vi "Initialize Scope and FGEN with Triggering.vi"(10 "FGEN Resources in":refnum<k15>[](array[refnum]), 11 "Scope Resources in":refnum<k15>[](array[refnum])) -> (0 "error out":errorcluster, 2 "FGEN Resources out":refnum<k15>[](array[refnum]), 3 "Scope Resources out":refnum<k15>[](array[refnum]), 5 "scope channels":string[](array[string]))   [LabVIEW 2024]
uses:
  <instrlib>/niFgen/niFgen.llb/niFgen Output Mode.ctl
  <instrlib>/niFgen/niFgen.llb/niFgen Trigger Mode.ctl
  <instrlib>/niScope/Controls/niScope input clock source.ctl
  <instrlib>/niScope/Controls/niScope trigger source digital.ctl
  <instrlib>/niScope/Controls/niScope trigger slope.ctl
  <instrlib>/niScope/Configure/Trigger/niScope Configure Trigger Digital.vi
  <instrlib>/niScope/Controls/niScope trigger source.ctl
  <instrlib>/niScope/Controls/niScope exportable signals.ctl
  <instrlib>/niScope/Controls/niScope export destinations.ctl
  <instrlib>/niScope/Configure/Trigger/niScope Configure Trigger Edge.vi
  <instrlib>/niFgen/niFgen.llb/niFgen_ctl Trigger Source Values (Ring).ctl
  <instrlib>/niFgen/niFgen.llb/niFgen Create Waveform (WDT).vi
  <instrlib>/niFgen/niFgen.llb/niFgen Configure Digital Edge Start Trigger.vi
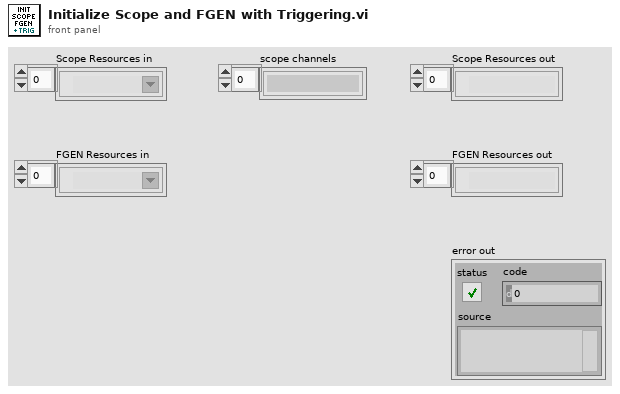
[diagram p1: front panel]
types:
  T1 = typedef "niFgen_ctl Trigger Source Values (Ring).ctl" = string
  T2 = typedef "niScope trigger source digital.ctl" = string
  T3 = typedef "niScope export destinations.ctl" = string
  T4 = typedef "niScope trigger source.ctl" = string
  T5 = typedef "niScope input clock source.ctl" = u16
  T6 = typedef "niScope trigger slope.ctl" = i32
  T7 = typedef "niScope exportable signals.ctl" = u16
  T8 = typedef "niFgen Trigger Mode.ctl" = i32
  T9 = typedef "niFgen Output Mode.ctl" = u32
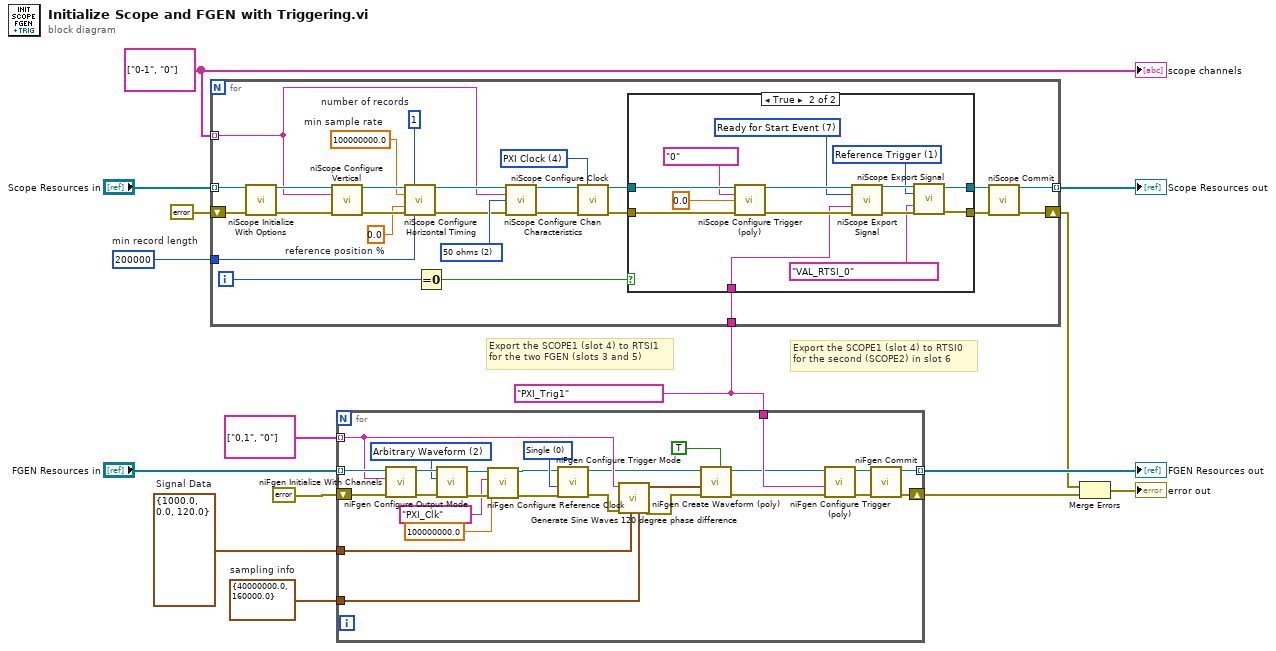
[diagram p0: block diagram]
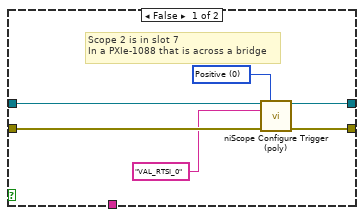
[diagram p2: hidden frame]
diagram:
  w15 = cluster{"f":dbl, "startPhase":dbl, "dPhase":dbl} {"f"=1000.0, "startPhase"=0.0, "dPhase"=120.0}  # Signal Data
  w14 = 200000  # min record length
  w11 = T1 "PXI_Trig1" ("Source")
  w10 = cluster{"Fs":dbl, "#s":dbl} {"Fs"=40000000.0, "#s"=160000.0}  # sampling info
  w6 = string[] ["0-1", "0"] ("channels")
  # "Export the SCOPE1 (slot 4) to RTSI0\nfor the second (SCOPE2) in slot 6"
  # "Export the SCOPE1 (slot 4) to RTSI1\nfor the two FGEN (slots 3 and 5)"
  n1 = for {
    tunnel: "Scope Resources in" -> [w30] mode=indexing
    tunnel: [w36] -> w3 mode=indexing
    tunnel: w6 -> [w17] mode=indexing
    shift-right: [w35] -> w1
    shift-left: errorcluster {"status"=FALSE, "code"=0, "source"=""} ("error out") -> [w34]
    tunnel: w11 -> [w26]
    tunnel: w14 -> [w16]
    i -> [w37]
    w22 = u32 2 items=["1 mega ohm"=0, "50 ohms"=2] ("input impedance")
    w23 = T5 4 items=["None"=0, "RTSI Clock"=1, "PFI 0"=6, "PFI 1"=2, "PFI 2"=3, "PXI Clock"=4, "External"=5, "Clock In"=7] ("input clock source")
    w31 = 0.0  # reference position %
    w32 = 1  # number of records
    w33 = 100000000.0  # min sample rate
    n2 = call <instrlib>:"niScope Initialize With Options.vi"("resource name"=w30, "error in"=w34) -> ("instrument handle"=w41:refnum<k15>, "error out"=w40:errorcluster)  [unwired: 12 in]
    n3 = call <instrlib>:"niScope Configure Vertical.vi"("instrument handle"=w41, "channels"=w17, "error in"=w40) -> ("instrument handle out"=w39:refnum<k15>, "error out"=w38:errorcluster)  [unwired: 11 in]
    n4 = call <instrlib>:"niScope Configure Horizontal Timing.vi"("instrument handle"=w39, "number of records"=w32, "min sample rate"=w33, "reference position"=w31, "error in"=w38, "min record length"=w16) -> ("instrument handle out"=w18:refnum<k15>, "error out"=w19:errorcluster)  [unwired: 8 in]
    n5 = Equal To 0?(x=w37) -> (x = 0?=w29:bool)
    n6 = call <instrlib>:"niScope Configure Chan Characteristics.vi"("instrument handle"=w18, "channels"=w17, "input impedance"=w22, "error in"=w19) -> ("instrument handle out"=w21:refnum<k15>, "error out"=w20:errorcluster)  [unwired: 10 in]
    n7 = call <instrlib>:"niScope Configure Clock.vi"("instrument handle"=w21, "input clock source"=w23, "error in"=w20) -> ("instrument handle out"=w24:refnum<k15>, "error out"=w25:errorcluster)  [unwired: 11 in]
    n8 = case shown="True" w29 {
      tunnel: w25 -> [w47 w60]
      tunnel: [w45 w51] -> w28
      tunnel: [w44 w52] -> w27
      tunnel: w24 -> [w46 w61]
      tunnel: w26 -> [_ w49]
      frame False {
        w42 = T6 0 items=["Positive", "Negative"] ("trigger slope")
        # "Scope 2 is in slot 7\nIn a PXIe-1088 that is across a bridge"
        n9 = call-poly <instrlib>:"niScope Configure Trigger (poly).vi"("instrument handle"=w46, "trigger slope"=w42, "trigger source"=T2 "VAL_RTSI_0", "error in"=w47) -> ("instrument handle out"=w45:refnum<k15>, "error out"=w44:errorcluster)  [unwired: 10 in]
      }
      frame True {
        w50 = T7 1 items=["None"=0, "Start Trigger"=2, "Advance Trigger"=5, "Reference Trigger"=1, "End of Record Event"=4, "End of Acquisition Event"=3, "Ready for Start Event"=7, "Ready for Advance Event"=6, "Ready for Reference Event"=10, "Reference Clock"=100, "Sample Clock"=101, "5 Volt Power"=13] ("signal")
        w55 = T7 7 items=["None"=0, "Start Trigger"=2, "Advance Trigger"=5, "Reference Trigger"=1, "End of Record Event"=4, "End of Acquisition Event"=3, "Ready for Start Event"=7, "Ready for Advance Event"=6, "Ready for Reference Event"=10, "Reference Clock"=100, "Sample Clock"=101, "5 Volt Power"=13] ("signal")
        n10 = call-poly <instrlib>:"niScope Configure Trigger (poly).vi"("instrument handle"=w61, "trigger source"=T4 "0", "trigger level"=0.0, "error in"=w60) -> ("instrument handle out"=w56:refnum<k15>, "error out"=w57:errorcluster)  [unwired: 10 in]
        n11 = call <instrlib>:"niScope Export Signal.vi"("instrument handle"=w56, "signal"=w55, "output terminal"=w49, "error in"=w57) -> ("instrument handle out"=w54:refnum<k15>, "error out"=w53:errorcluster)  [unwired: 10 in]
        n12 = call <instrlib>:"niScope Export Signal.vi"("instrument handle"=w54, "signal"=w50, "output terminal"=T3 "VAL_RTSI_0", "error in"=w53) -> ("instrument handle out"=w51:refnum<k15>, "error out"=w52:errorcluster)  [unwired: 10 in]
      }
    }
    n13 = call <instrlib>:"niScope Commit.vi"("instrument handle"=w28, "error in"=w27) -> ("instrument handle out"=w36:refnum<k15>, "error out"=w35:errorcluster)  [unwired: 12 in]
  }
  "Scope Resources out" <- w3
  n14 = for {
    tunnel: "FGEN Resources in" -> [w85] mode=indexing
    tunnel: [w88] -> w12 mode=indexing
    tunnel: string[] ["0,1", "0"] ("channels") -> [w72] mode=indexing
    shift-right: [w87] -> w4
    shift-left: errorcluster {"status"=FALSE, "code"=0, "source"=""} ("error out") -> [w86]
    tunnel: w10 -> [w70]
    tunnel: w11 -> [w77]
    tunnel: w15 -> [w71]
    w80 = T8 0 items=["Single", "Continuous", "Stepped", "Burst"] ("Trigger Mode (default: 1=continuous)")
    w82 = T9 2 items=["Standard Function", "Frequency List", "Arbitrary Waveform", "Arbitrary Sequence", "Script"] ("Output Mode (default: 0=Standard Function)")
    n15 = call <instrlib>:"niFgen Initialize With Channels.vi"("error in (no error)"=w86, "Channel Name"=w72, "Resource Name"=w85) -> ("error out"=w84:errorcluster, "Instrument Handle Out"=w83:refnum<k15>)  [unwired: 7 in]
    n16 = call <instrlib>:"niFgen Configure Output Mode.vi"("error in (no error)"=w84, "Output Mode (default: 0=Standard Function)"=w82, "Instrument Handle"=w83) -> ("error out"=w76:errorcluster, "Instrument Handle Out"=w75:refnum<k15>)  [unwired: 6 in]
    n17 = call <instrlib>:"niFgen Configure Reference Clock.vi"("error in (no error)"=w76, "Reference Clock Frequency"=100000000.0, "Source"="PXI_Clk", "Instrument Handle"=w75) -> ("error out"=w67:errorcluster, "Instrument Handle Out"=w66:refnum<k15>)  [unwired: 6 in]
    n18 = call <instrlib>:"niFgen Configure Trigger Mode.vi"("error in (no error)"=w67, "Trigger Mode (default: 1=continuous)"=w80, "Instrument Handle"=w66) -> ("error out"=w64:errorcluster, "Instrument Handle Out"=w65:refnum<k15>)  [unwired: 7 in]
    n19 = call "Generate Sine Waves 120 degree phase difference.vi"("sampling info"=w70, "Signal Data"=w71, "error in (no error)"=w64, "channels"=w72) -> ("error out"=w68:errorcluster, "signal out"=w69:waveform(dbl))  [unwired: 6 in]
    n20 = call-poly <instrlib>:"niFgen Create Waveform (poly).vi"("Use Waveform dT for Sample Rate"=TRUE, "error in (no error)"=w68, "Waveform"=w69, "Instrument Handle"=w65) -> ("error out"=w63:errorcluster, "Instrument Handle Out"=w62:refnum<k15>)  [unwired: 5 in, 1 out]
    n21 = call-poly <instrlib>:"niFgen Configure Trigger (poly).vi"("error in (no error)"=w63, "Source"=w77, "Instrument Handle"=w62) -> ("error out"=w78:errorcluster, "Instrument Handle Out"=w79:refnum<k15>)  [unwired: 7 in]
    n22 = call <instrlib>:"niFgen Commit.vi"("error in (no error)"=w78, "Instrument Handle"=w79) -> ("error out"=w87:errorcluster, "Instrument Handle Out"=w88:refnum<k15>)  [unwired: 8 in]
  }
  "FGEN Resources out" <- w12
  n23 = Merge Errors(w1, w4) -> (→"error out":errorcluster)
  "scope channels" <- w6
